vi "set_params.vi"(0 "dummyStageRapid in":refnum<class "dummyStageRapid.lvclass">, 3 "error in (no error)":errorcluster) -> (7 "dummyStageRapid out":refnum<class "dummyStageRapid.lvclass">, 10 "error out":errorcluster)   [LabVIEW 2019, in "dummyStageRapid.lvlib" / "dummyStageRapid.lvclass"]
uses:
  dummyStageRapid.lvclass
panel:
  in  "pos_max":dbl[](array[numeric])=[10000.0]
  in  "OK Button":bool
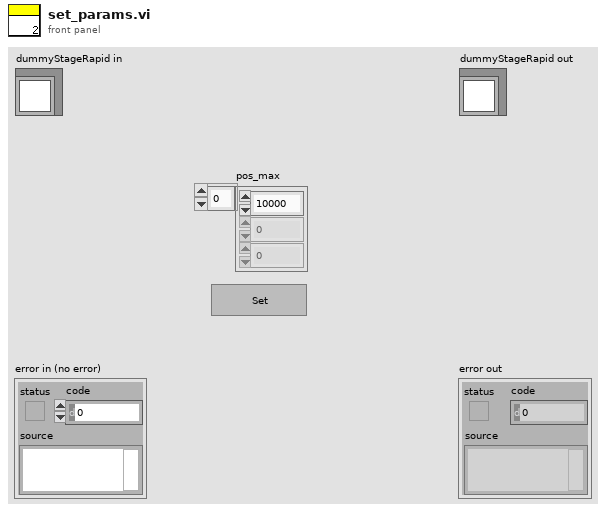
[diagram p1: front panel]
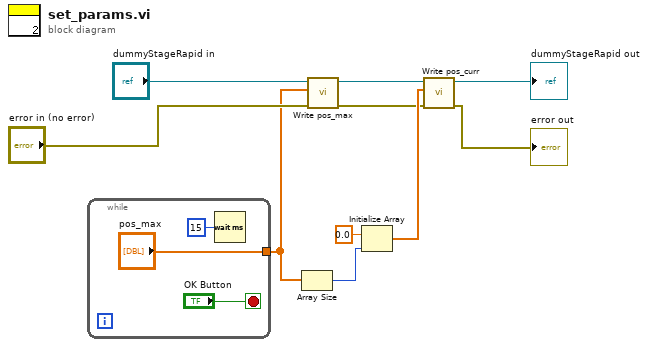
[diagram p0: block diagram]
diagram:
  n1 = while {
    tunnel: ["pos_max"] -> w4
    stop <- "OK Button" stop-if-true
    n2 = Wait (ms)(milliseconds to wait=u32 15) -> ()  [unwired: 1 out]
  }
  n3 = Array Size(array=w4) -> (size(s)=w5:i32)
  n4 = call-dynamic "Write pos_max.vi"("error in (no error)"="error in (no error)", "pos_max"=w4, "_stage in"="dummyStageRapid in") -> ("error out"=w2:errorcluster, "_stage out"=w9:refnum<class "dummyStageRapid.lvclass">)  [unwired: 7 in]
  n5 = Initialize Array(0.0 ("element"), w5) -> (w3:dbl[])
  n6 = call-dynamic "Write pos_curr.vi"("error in (no error)"=w2, "set_pos"=w3, "_stage in"=w9) -> ("error out"=→"error out":errorcluster, "_stage out"=→"dummyStageRapid out":refnum<class "dummyStageRapid.lvclass">)  [unwired: 7 in]
